vi "zmq ctx shutdown.vi"(8 "error in (no error)":errorcluster, 11 "context_":u32) -> (0 "error out":errorcluster, 2 "function return":i32, 3 "context_ out":u32)   [LabVIEW 2025, in "libzmq-v143-mt-4_3_6.lvlib"]
doc: "ZMQ_EXPORT int zmq_ctx_shutdown (void *context_);"
uses:
  libzmq-v143-mt-4_3_6.lvlib
  LV/LibZMQ/libzmq/lv_x86/bin/Release/libzmq-v143-mt-4_3_6.dll
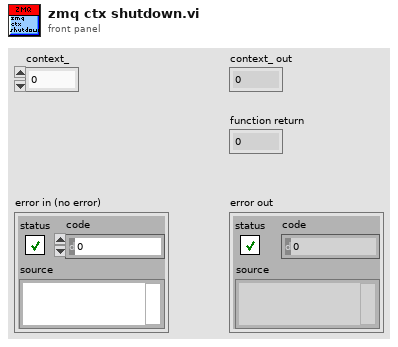
[diagram p1: front panel]
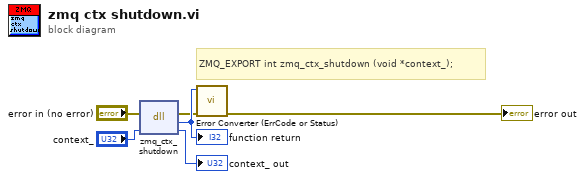
[diagram p0: block diagram]
diagram:
  # "ZMQ_EXPORT int zmq_ctx_shutdown (void *context_);"
  n1 = dll-call lib="C:/LV/LibZMQ/libzmq/lv_x86/bin/Release/libzmq-v143-mt-4_3_6.*" fn="zmq_ctx_shutdown"(error in="error in (no error)", "context_"="context_") -> (error out=w2:errorcluster, w6:i32, "context_"=→"context_ out":u32)  [unwired: 2 in, 1 out]
  "function return" <- w6
  n2 = call "Error Converter (ErrCode or Status).vi"("error in (no error)"=w2, "error code"=w6) -> ("error out"=→"error out":errorcluster)  [unwired: 9 in]
